vi "Open.vi"(8 "error in (no error)":errorcluster, 11 "Modbus in":refnum<class "Modbus.lvclass">) -> (0 "error out":errorcluster, 3 "Modbus out":refnum<class "Modbus.lvclass">)   [LabVIEW 2018, in "Modbus.lvclass"]
doc: "Modbus.lvclass:Open.vi\n\nThis VI opens a connection for the Modbus communications.\n\nInstrument Communication Module Version 1.0\nJanuary, 2017 Original Code Consulting David Thomson\n www.originalcode.com"
uses:
  Modbus.lvclass
  Modbus.lvclass/Modbus.ctl
  <vilib>/Modbus/subvis/Modbus API/Modbus API.lvclass/Modbus API.ctl
  <vilib>/Modbus/subvis/Transmission Data Unit (ADU)/Transmission Data Unit/Transmission Data Unit.lvclass/Transmission Data Unit.ctl
  <vilib>/Modbus/master/Data Access/Unit ID/Set Unit ID Property.vi
  <vilib>/Modbus/subvis/Transmission Data Unit (ADU)/Transmission Data Unit/Data Access/Unit ID/Write Unit ID.vi
  <vilib>/Modbus/subvis/Modbus API/Read Transmission Data Unit.vi
  <vilib>/Modbus/subvis/Modbus API/Write Transmission Data Unit.vi
  <vilib>/Modbus/master/Modbus Master.lvclass
  C:/Program Files (x86)/National Instruments/LabVIEW 2018/vi.lib/Modbus/subvis/Modbus API/Modbus API.lvclass
  <vilib>/Modbus/master/Create Master Instance (TCP).vi
  <vilib>/Modbus/master/Create Master Instance (Serial).vi
  <vilib>/Modbus/subvis/Transmission Data Unit (ADU)/Transmission Data Unit/Transmission Data Unit.lvclass
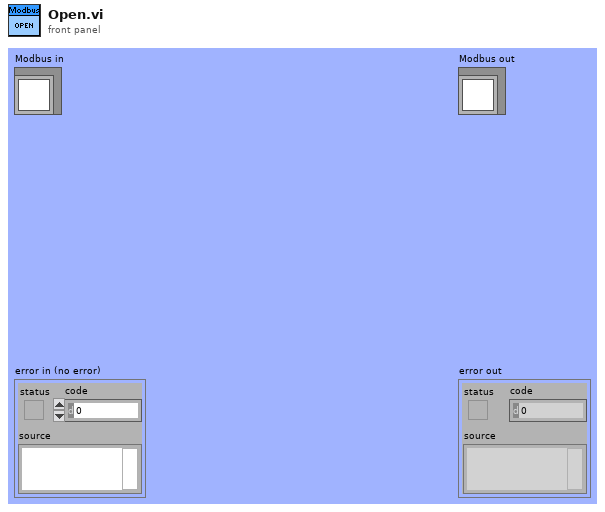
[diagram p1: front panel]
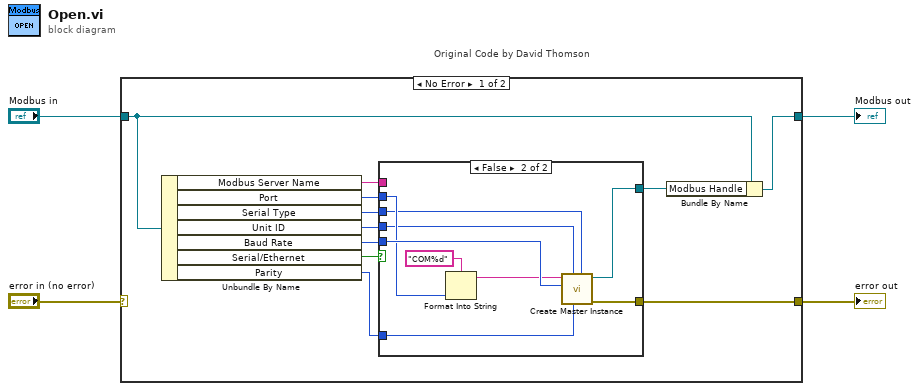
[diagram p0: block diagram]
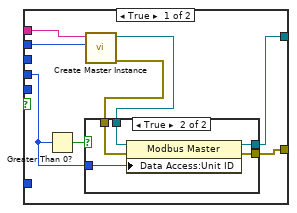
[diagram p2: hidden frame]
diagram:
  n1 = case "Original Code by David Thomson" shown="No Error" "error in (no error)" {
    selector: "error in (no error)" -> [_ w41]
    tunnel: [w5 w41] -> w3
    tunnel: "Modbus in" -> [w8 w40]
    tunnel: [w6 w40] -> w1
    frame No Error {
      n2 = Unbundle By Name(w8) -> ("Modbus Server Name"=w11:string, "Port"=w10:u16, "Serial Type"=w12:enum16{"RTU", "ASCII"}, "Unit ID"=w13:u8, "Baud Rate"=w14:u32, "Serial/Ethernet"=w15:bool, "Parity"=w9:u16)
      n3 = case shown="False" w15 {
        tunnel: w11 -> [w23 _]
        tunnel: [w18 w39] -> w5
        tunnel: [w19 w38] -> w7
        tunnel: w10 -> [w22 w36]
        tunnel: w14 -> [_ w37]
        tunnel: w12 -> [_ w34]
        tunnel: w13 -> [w16 w33]
        tunnel: w9 -> [_ w31]
        frame True {
          n4 = Greater Than 0?(x=w16) -> (x > 0?=w17:bool)
          n5 = call-poly <vilib>:"Create Master Instance.vi"("port (502)"=w22, "address"=w23) -> ("error out"=w20:errorcluster, "TCP master instance"=w21:refnum<class "Modbus Master.lvclass">)  [unwired: 8 in]
          n6 = case shown="True" w17 {
            tunnel: w21 -> [w24 w30]
            tunnel: w20 -> [w25 w29]
            tunnel: [w24 w28] -> w19
            tunnel: [w25 w27] -> w18
            tunnel: w16 -> [_ w26]
            frame False {
            }
            frame True {
              n7 = property class="Modbus Master"(reference=w30, error in=w29, "Data Access:Unit ID"=w26) -> (reference out=w28:refnum<class "Modbus Master.lvclass">, error out=w27:errorcluster)
            }
          }
        }
        frame False {
          n8 = Format Into String(format string="COM%d", w36) -> (resulting string=w32:string)  [unwired: 2 in, 1 out]
          n9 = call-poly <vilib>:"Create Master Instance.vi"("serial type"=w34, "parity (Even)"=w31, "unit ID"=w33, "baud rate (9600)"=w37, "VISA resource name"=w32) -> ("error out"=w39:errorcluster, "serial master instance"=w38:refnum<class "Modbus Master.lvclass">)  [unwired: 5 in]
        }
      }
      n10 = Bundle By Name(cluster=w8, "Modbus Handle"=w7) -> (w6:refnum<class "Modbus.lvclass">)
    }
    frame Error {
    }
  }
  "error out" <- w3
  "Modbus out" <- w1
